vi "Add View.vi"(0 "Controller in":refnum<class "Controller.lvclass">, 1 "View Actor":refnum<class "View.lvclass">, 2 "Exclude From Broadcast (F)":bool, 3 "Paused (F)":bool, 4 "Receive Only (F)":bool, 5 "error in (no error)":errorcluster) -> (14 "Controller out":refnum<class "Controller.lvclass">, 16 "View Enqueuer":refnum<class "Message Enqueuer.lvclass">, 19 "error out":errorcluster)   [LabVIEW 2023, in "MVC Actors.lvlib" / "Controller.lvclass"]
doc: "Starts a View Actor with following settings:\n\n<b>Exclude From Broadcast</b>: message originating form another view will not be broadcasted to the view being cosidered\n<b>Paused</b>: the view will not send events and will not receive them anymore\n<b>Receive only</b>: The view will receive events but not send any"
uses:
  Controller.lvclass
  C:/Program Files/National Instruments/LabVIEW 2023/vi.lib/ActorFramework/Actor/Actor.lvclass
  View/View.lvclass
  <vilib>/ActorFramework/Message Enqueuer/Message Enqueuer.lvclass
  View Details.ctl
  View/View.lvclass/View.ctl
  Controller.lvclass/Controller.ctl
  <vilib>/ActorFramework/Actor/Actor.lvclass/Actor.ctl
  <vilib>/ActorFramework/Message Enqueuer/Message Enqueuer.lvclass/Message Enqueuer.ctl
  View Messages/Write Controller Actor Enqueuer Msg/Write Controller Actor Enqueuer Msg.lvclass/Write Controller Actor Enqueuer Msg.ctl
  View/properties/Read Name.vi
  View/properties/Write Paused.vi
  View/properties/Write Receive Only.vi
  <vilib>/ActorFramework/Message Enqueuer/Init from Existing Queue.vi
  <vilib>/ActorFramework/Message Enqueuer/Enqueue.vi
  View Messages/Write Controller Actor Enqueuer Msg/Write Controller Actor Enqueuer Msg.lvclass
  C:/Program Files/National Instruments/LabVIEW 2023/vi.lib/ActorFramework/Message/Message.lvclass
  <vilib>/Utility/LVClass/Get LV Class Name.vi
  <resource>/AFDebug/Generate Trace for Message.vi
  <vilib>/ActorFramework/Message Priority Queue/Priority Enqueue.vi
  <vilib>/ActorFramework/Actor/Actor.lvclass
  C:/Program Files/National Instruments/LabVIEW 2023/vi.lib/LS Instruments AG/Async Methods Actor/Async Methods Actor/Async Methods Actor/Async Methods Actor.lvclass
  C:/Projects/Shared Libraries/Event Actors/Controller/Controller.lvclass
  C:/Projects/Shared Libraries/Event Actors/View/View.lvclass
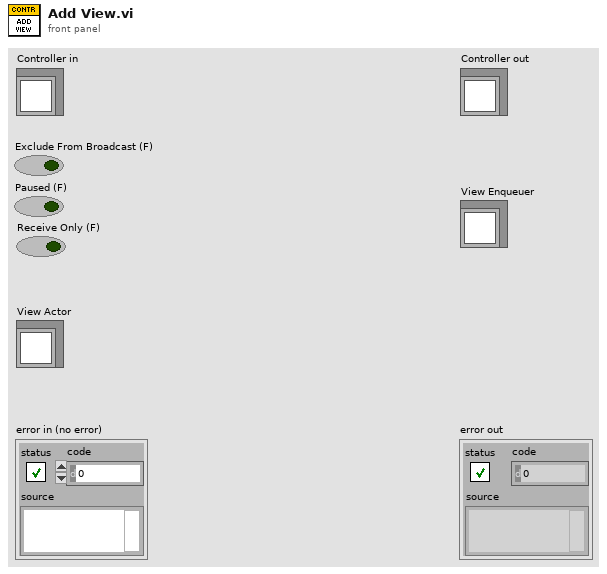
[diagram p1: front panel]
types:
  T1 = typedef "MVC Actors.lvlib/Controller.lvclass/View Details.ctl" = cluster{"Exclude From Broadcast":bool, "Receive Only":bool, "Paused":bool, "View Enqueuer":refnum<class "Message Enqueuer.lvclass">}
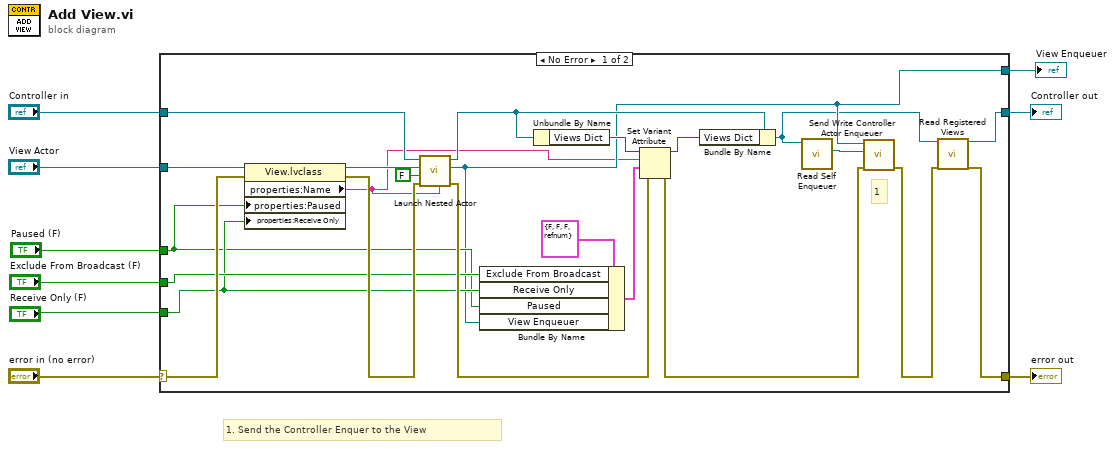
[diagram p0: block diagram]
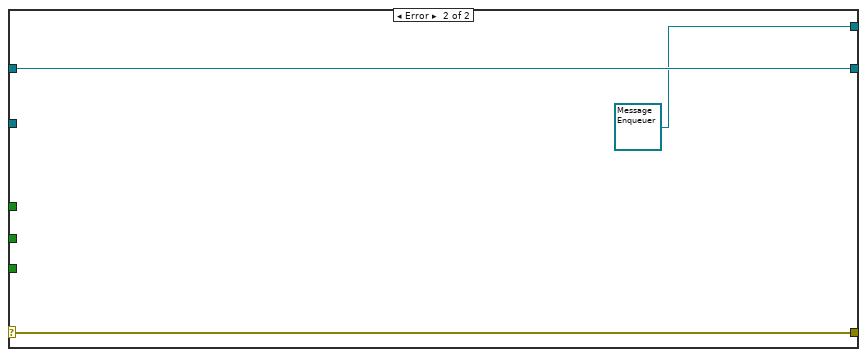
[diagram p2: hidden frame]
diagram:
  # "1. Send the Controller Enquer to the View"
  n1 = case shown="No Error" "error in (no error)" {
    selector: "error in (no error)" -> [w24 w35]
    tunnel: [w12 w35] -> w8
    tunnel: [w10 w34] -> w6
    tunnel: "Controller in" -> [w28 w34]
    tunnel: "View Actor" -> [w29 _]
    tunnel: "Paused (F)" -> [w16 _]
    tunnel: "Exclude From Broadcast (F)" -> [w18 _]
    tunnel: "Receive Only (F)" -> [w17 _]
    tunnel: [w15 refnum<class "Message Enqueuer.lvclass"> refnum ("Nested Actor's Enqueuer")] -> w1
    frame No Error {
      # "1"
      n2 = property class="View.lvclass"(reference=w29, error in=w24, "properties:Paused"=w16, "properties:Receive Only"=w17) -> (reference out=w25:refnum<class "View.lvclass">, error out=w23:errorcluster, "properties:Name"=w14:string)
      n3 = call <vilib>:"Launch Nested Actor.vi"("Debug Alias"=w14, "error in (no error)"=w23, "Auto-stop? (T)"=FALSE, "Nested Actor"=w25, "Caller Actor in"=w28) -> ("error out"=w30:errorcluster, "Nested Actor's Enqueuer"=w15:refnum<class "Message Enqueuer.lvclass">, "Caller Actor out"=w27:refnum<class "Controller.lvclass">)  [unwired: 4 in]
      n4 = Bundle By Name(cluster=T1 {"Exclude From Broadcast"=FALSE, "Receive Only"=FALSE, "Paused"=FALSE, "View Enqueuer"=refnum} ("Sink Settings"), "Exclude From Broadcast"=w18, "Receive Only"=w17, "Paused"=w16, "View Enqueuer"=w15) -> (w19:T1)
      n5 = Unbundle By Name(w27) -> ("Views Dict"=w32:variant)
      n6 = Set Variant Attribute(Variant=w32, name=w14, value=w19, error in=w30) -> (Variant out=w31:variant, error out=w21:errorcluster)  [unwired: 1 out]
      n7 = Bundle By Name(cluster=w27, "Views Dict"=w31) -> (w11:refnum<class "Controller.lvclass">)
      n8 = call <vilib>:"Read Self Enqueuer.vi"("Actor"=w11) -> ("Self Enqueuer"=w22:refnum<class "Message Enqueuer.lvclass">)  [unwired: 10 in]
      n9 = call "Send Write Controller Actor Enqueuer.vi"("error in (no error)"=w21, "Controller Actor Enqueuer"=w22, "Message Enqueuer in"=w15) -> ("error out"=w13:errorcluster)  [unwired: 7 in, 1 out]
      n10 = call "Read Registered Views.vi"("Controller in"=w11, "error in (no error)"=w13) -> ("Controller out"=w10:refnum<class "Controller.lvclass">, "error out"=w12:errorcluster)  [unwired: 16 in]
    }
    frame Error {
    }
  }
  "error out" <- w8
  "Controller out" <- w6
  "View Enqueuer" <- w1
